vi "main.vi"() -> ()   [LabVIEW 2019]
uses:
  <vilib>/Analysis/3filter.llb/Filter Passband Type.ctl
  <vilib>/addons/control/pid/autopid.llb/PID autotuning parameters (FO).ctl
  <vilib>/Analysis/3filter.llb/Butterworth Filter (DBL).vi
  <vilib>/addons/control/pid/NI_PID_autopid.lvlib
  <vilib>/Analysis/NI_AALBase.lvlib
panel:
  in  "fine-tuning threshold (degreeC)":dbl format="%#_13g"
  in  "fine-tuning voltage (V)":dbl format="%#_13g"
  in  "limiting current (A)":dbl format="%#_13g"
  in  "heating voltage (V)":dbl format="%#_13g"
  out "Running?":bool
  in  "Graph Tab":T1(tab)
  out "Temperature Difference (sample - ambient)":cluster{dbl[], dbl[]}(graph)
  out "Temperature":cluster{dbl[], dbl[]}[](graph)
  out "Transient Power":cluster{dbl[], dbl[]}(graph)
  out "Current":cluster{dbl[], dbl[]}(graph)
  out "Voltage":cluster{dbl[], dbl[]}(graph)
  out "compensation":dbl(graph)
  out "Vp":dbl(graph)
  in  "display duration (s)":dbl format="%#_13g"
  in  "sampling interval (s)":dbl format="%#_13g"
  in  "pld_3605":refnum<visa-resource-name>
  in  "keithley_6510":refnum<visa-resource-name>
  in  "Stop Button":bool
  in  "Run Button":bool
  # "white: sample, red: ambient"
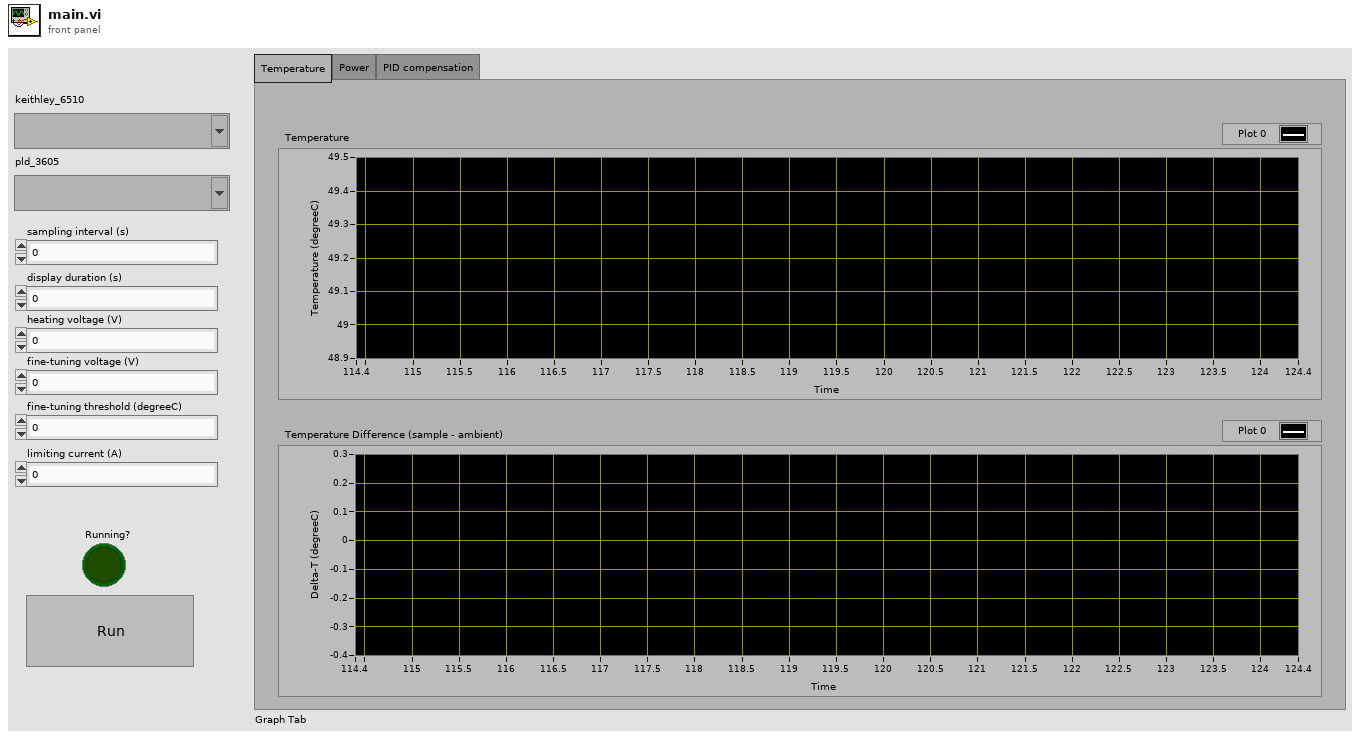
[diagram p1: front panel]
types:
  T1 = enum32{"Temperature", "Power", "PID compensation"}
  T2 = enum8{"Enabled", "Disabled", "Disabled and Grayed Out"}
  T3 = enum16{"open", "replace", "create", "open or create", "replace or create", "replace or create with confirmation"}
  T4 = cluster{"proportional gain (Kc)":dbl, "integral time (Ti, min)":dbl, "derivative time (Td, min)":dbl}
  T5 = typedef "NI_PID_autopid.lvlib/PID autotuning parameters (FO).ctl" = cluster{"type of controller":u16, "time constant factor":dbl, "step amplitude":dbl}
  T6 = typedef "NI_AALBase.lvlib/Filter Passband Type.ctl" = enum32{"Lowpass", "Highpass", "Bandpass", "Bandstop"}
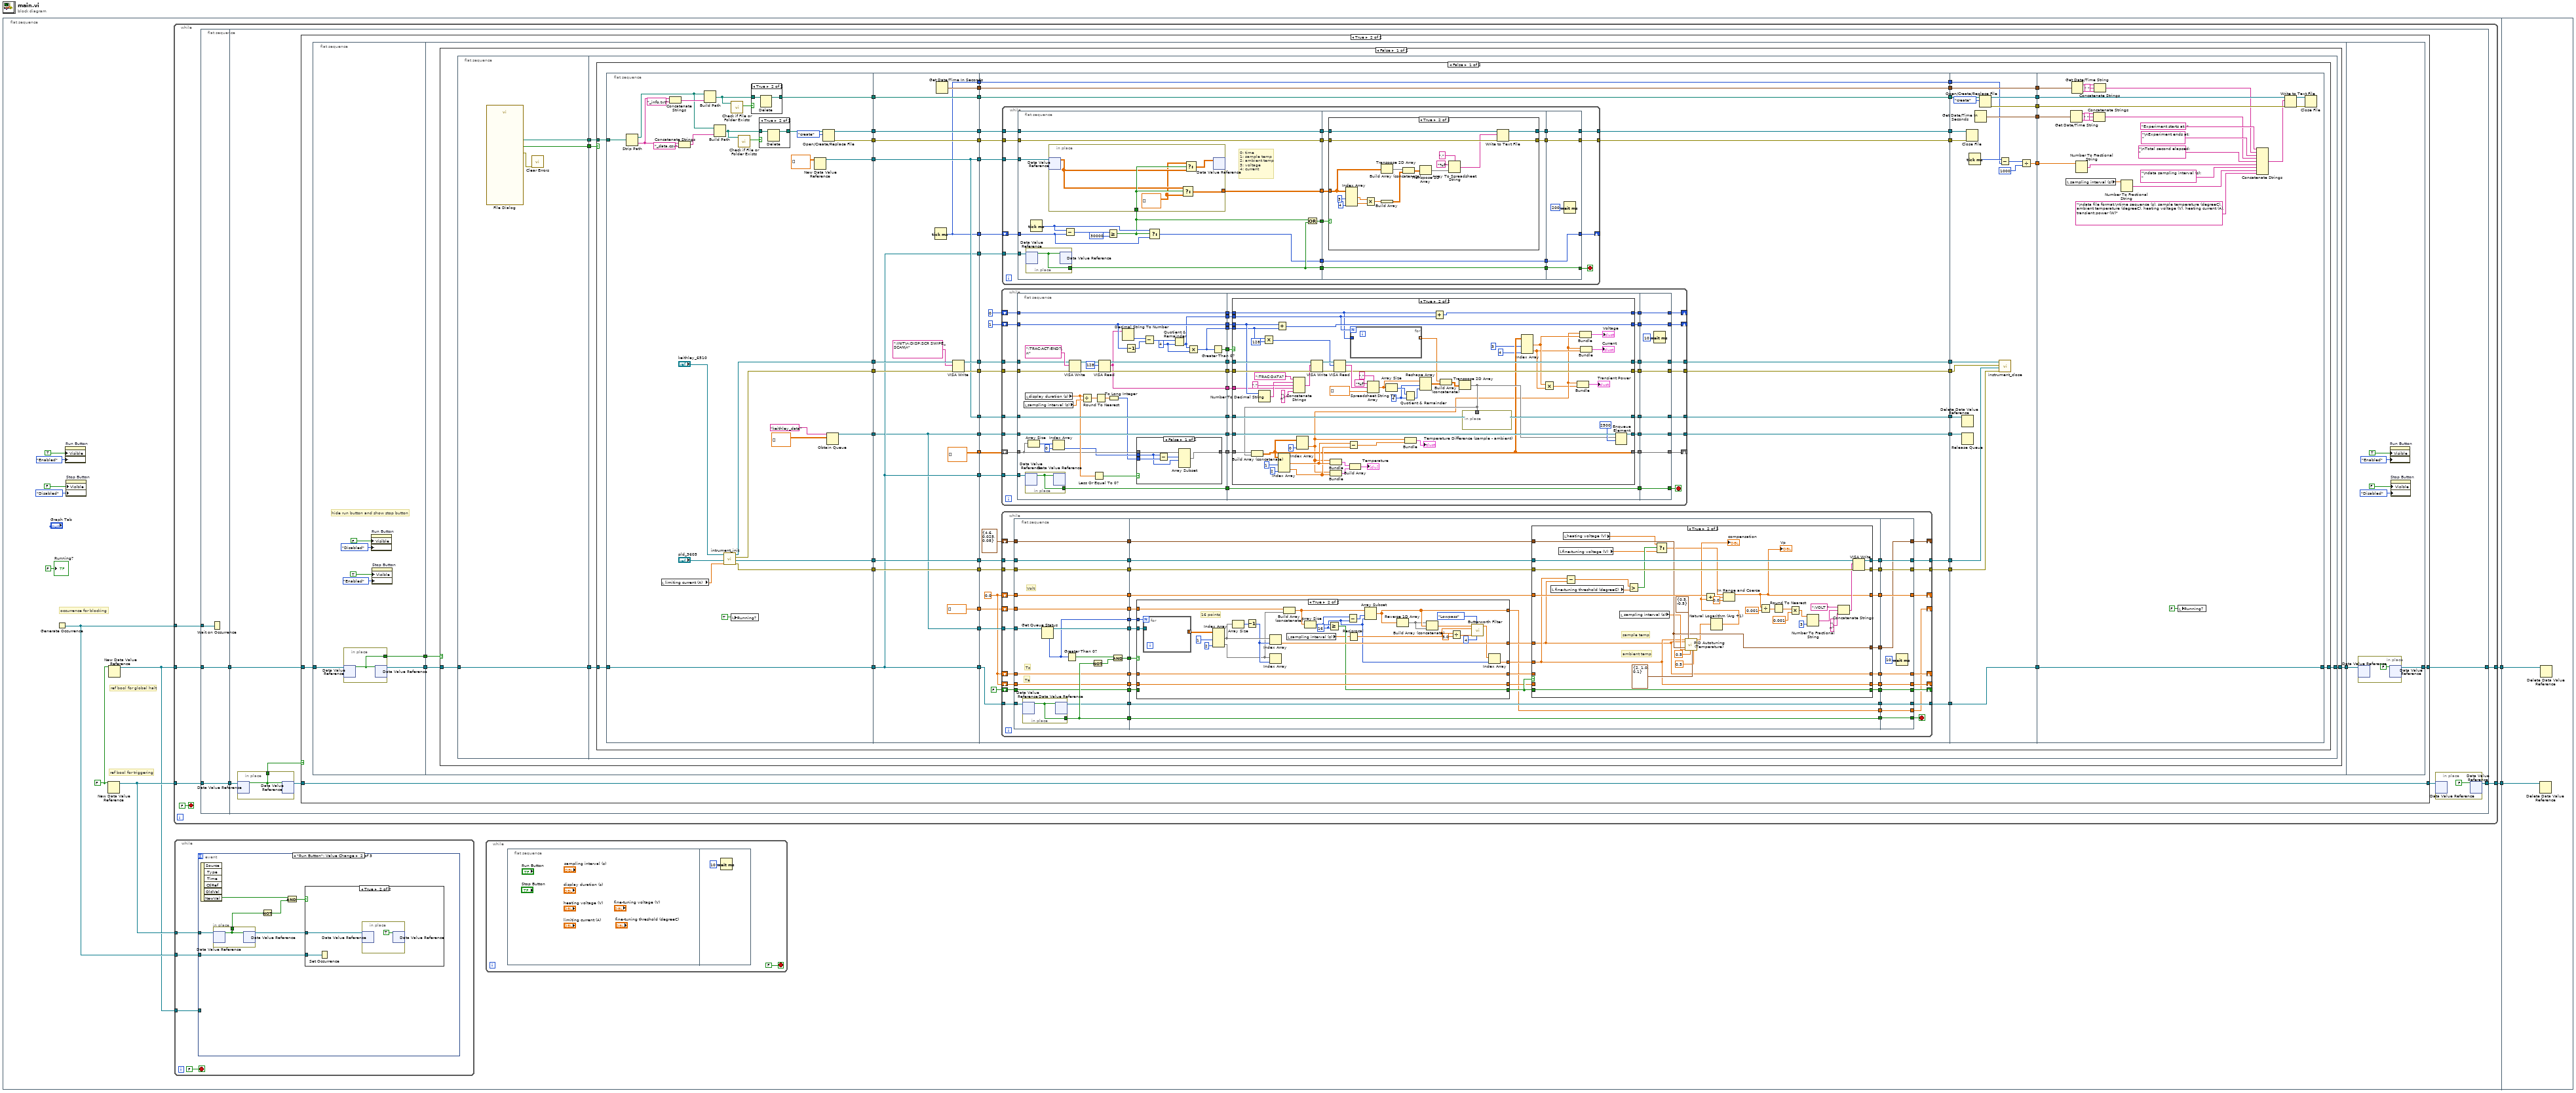
[diagram p0: block diagram]
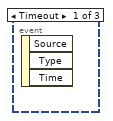
[diagram p2: hidden frame]
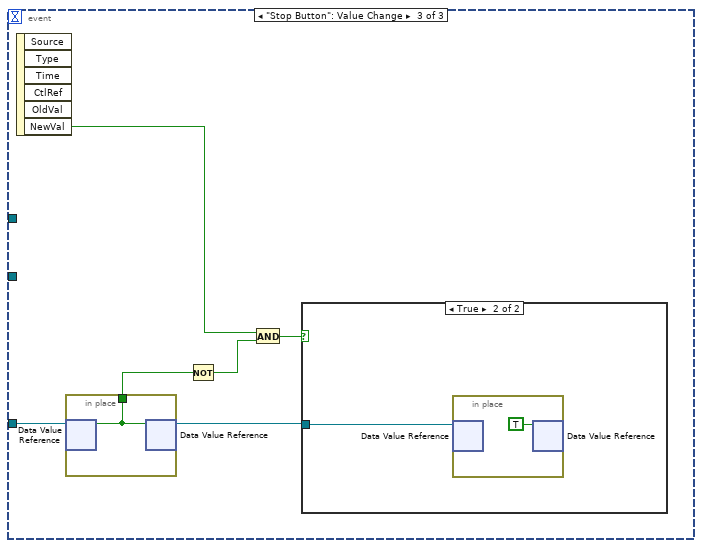
[diagram p4: hidden frame]
diagram:
  n1 = flat-sequence {
    tunnel: [w9] -> w2
    tunnel: [w8] -> w1
    tunnel: w2 -> [w706]
    tunnel: w1 -> [w705]
    frame #0 {
      w12 = FALSE
      # "occurrence for blocking"
      # "ref bool for global halt"
      # "ref bool for triggering"
      n2 = Generate Occurrence() -> (w11:refnum<k4>)
      n3 = property on="Run Button" class="Bool"("Visible"=TRUE, "DisabledEnum"=T2."Enabled" ("Disabled")) -> ()  [unwired: 2 in, 2 out]
      n4 = property on="Stop Button" class="Bool"("Visible"=FALSE, "DisabledEnum"=T2."Disabled" ("Disabled")) -> ()  [unwired: 2 in, 2 out]
      n5 = New Data Value Reference(data value=w12) -> (data value reference=w13:refnum<data-value>)  [unwired: 1 in, 1 out]
      n6 = New Data Value Reference(data value=w12) -> (data value reference=w10:refnum<data-value>)  [unwired: 1 in, 1 out]
      n7 = while {
        tunnel: w13 -> [w45]
        tunnel: w10 -> [w43]
        tunnel: w11 -> [w42]
        tunnel: [w41] -> w9
        tunnel: [w40] -> w8
        stop <- FALSE stop-if-true
        n8 = flat-sequence {
          tunnel: [w50] -> w46
          tunnel: w45 -> [w50]
          tunnel: [w49] -> w44
          tunnel: w43 -> [w49]
          tunnel: w42 -> [w48]
          tunnel: w46 -> [w57]
          tunnel: w44 -> [w55]
          tunnel: [w52] -> w41
          tunnel: [w51] -> w40
          frame #0 {
            n9 = Wait on Occurrence(2:w48) -> ()  [unwired: 2 in, 1 out]
          }
          frame #1 {
            n10 = in-place {
              in-place-border: [w59] -> w56
              n11 = in-place-dvr #1(w57) -> (w59:bool)  [unwired: 1 out]
              n12 = in-place-dvr #1(w59) -> (w54:refnum<data-value>)  [unwired: 1 out]
            }
            n13 = case shown="True" w56 {
              tunnel: w55 -> [w60 w67]
              tunnel: w54 -> [w61 w63]
              tunnel: [w61 w63] -> w53
              tunnel: [w60 w62] -> w52
              frame False {
              }
              frame True {
                n14 = flat-sequence {
                  tunnel: w67 -> [w74]
                  tunnel: [w73] -> w66
                  tunnel: [w72] -> w65
                  tunnel: w66 -> [w78]
                  tunnel: w65 -> [w77]
                  tunnel: [w76] -> w64
                  tunnel: w64 -> [w703]
                  tunnel: [w702] -> w62
                  frame #0 {
                    # "hide run button and show stop button"
                    n15 = in-place {
                      in-place-border: [w75] -> w72
                      n16 = in-place-dvr #2(w74) -> (w75:bool)  [unwired: 1 out]
                      n17 = in-place-dvr #2(w75) -> (w73:refnum<data-value>)  [unwired: 1 out]
                    }
                    n18 = property on="Run Button" class="Bool"("Visible"=FALSE, "DisabledEnum"=T2."Disabled" ("Disabled")) -> ()  [unwired: 2 in, 2 out]
                    n19 = property on="Stop Button" class="Bool"("Visible"=TRUE, "DisabledEnum"=T2."Enabled" ("Disabled")) -> ()  [unwired: 2 in, 2 out]
                  }
                  frame #1 {
                    n20 = case shown="False" w77 {
                      tunnel: w78 -> [w80 w697]
                      tunnel: [w79 w697] -> w76
                      frame False {
                        n21 = flat-sequence {
                          tunnel: [w86] -> w83
                          tunnel: [w85] -> w82
                          tunnel: [w84] -> w81
                          tunnel: w80 -> [w84]
                          tunnel: w83 -> [w91]
                          tunnel: w82 -> [w90]
                          tunnel: w81 -> [w89]
                          tunnel: [w88] -> w79
                          frame #0 {
                            n22 = call "File Dialog"() -> ("selected path"=w85:path, "cancelled"=w86:bool, "error out"=w87:errorcluster)  [unwired: 12 in, 1 out]
                            n23 = call <vilib>:"Clear Errors.vi"("error in (no error)"=w87) -> ()  [unwired: 5 in, 2 out]
                          }
                          frame #1 {
                            n24 = case shown="False" w91 {
                              tunnel: w90 -> [w141 _]
                              tunnel: w89 -> [w128 w696]
                              tunnel: [w106 w696] -> w88
                              frame False {
                                n25 = flat-sequence {
                                tunnel: w141 -> [w161]
                                tunnel: [w169] -> w139
                                tunnel: [w168] -> w138
                                tunnel: [w167] -> w137
                                tunnel: [w166] -> w136
                                tunnel: [w155] -> w135
                                tunnel: [w152] -> w133
                                tunnel: [w151] -> w132
                                tunnel: [w149] -> w131
                                tunnel: w128 -> [w148]
                                tunnel: [w148] -> w127
                                tunnel: [w145] -> w117
                                tunnel: [w193] -> w140
                                tunnel: w139 -> [w190]
                                tunnel: w138 -> [w184]
                                tunnel: w137 -> [w189]
                                tunnel: w136 -> [w183]
                                tunnel: w135 -> [w194]
                                tunnel: [w194] -> w134
                                tunnel: w133 -> [w192]
                                tunnel: w132 -> [w191]
                                tunnel: w131 -> [w185]
                                tunnel: [w192] -> w130
                                tunnel: [w191] -> w129
                                tunnel: w127 -> [w182]
                                tunnel: [w182] -> w126
                                tunnel: [w185] -> w125
                                tunnel: [w179] -> w124
                                tunnel: [w187] -> w123
                                tunnel: [w186] -> w122
                                tunnel: [w182] -> w121
                                tunnel: [w185] -> w118
                                tunnel: w117 -> [w181]
                                tunnel: [w181] -> w116
                                tunnel: [w184] -> w113
                                tunnel: [w183] -> w112
                                tunnel: [w182] -> w111
                                tunnel: [w181] -> w110
                                tunnel: [dbl[][] []] -> w96
                                tunnel: [w179] -> w95
                                tunnel: [dbl[] []] -> w92
                                tunnel: w140 -> [w200]
                                tunnel: w134 -> [w199]
                                tunnel: w130 -> [w227]
                                tunnel: w129 -> [w226]
                                tunnel: w126 -> [w225]
                                tunnel: w125 -> [w224]
                                tunnel: w124 -> [w223]
                                tunnel: w123 -> [w222]
                                tunnel: w122 -> [w221]
                                tunnel: w121 -> [w220]
                                tunnel: [w217] -> w120
                                tunnel: [w216] -> w119
                                tunnel: w118 -> [w215]
                                tunnel: w116 -> [w214]
                                tunnel: [w213] -> w115
                                tunnel: [w212] -> w114
                                tunnel: w113 -> [w211]
                                tunnel: w112 -> [w210]
                                tunnel: w111 -> [w209]
                                tunnel: w110 -> [w208]
                                tunnel: [w207] -> w109
                                tunnel: [w206] -> w108
                                tunnel: [w203] -> w107
                                tunnel: [w202] -> w104
                                tunnel: [w201] -> w103
                                tunnel: [w200] -> w102
                                tunnel: [w199] -> w101
                                tunnel: w96 -> [w198]
                                tunnel: w95 -> [w197]
                                tunnel: [w197] -> w94
                                tunnel: w92 -> [w195]
                                tunnel: w120 -> [w667]
                                tunnel: w119 -> [w666]
                                tunnel: w115 -> [w668]
                                tunnel: w114 -> [w669]
                                tunnel: w109 -> [w665]
                                tunnel: w108 -> [w664]
                                tunnel: w107 -> [w663]
                                tunnel: [w663] -> w105
                                tunnel: w104 -> [w662]
                                tunnel: w103 -> [w661]
                                tunnel: w102 -> [w659]
                                tunnel: w101 -> [w658]
                                tunnel: [w660] -> w100
                                tunnel: [w659] -> w99
                                tunnel: [w656] -> w98
                                tunnel: [w655] -> w97
                                tunnel: w94 -> [w653]
                                tunnel: [w650] -> w93
                                tunnel: [w695] -> w106
                                tunnel: w105 -> [w695]
                                tunnel: w100 -> [w683]
                                tunnel: w99 -> [w689]
                                tunnel: w98 -> [w694]
                                tunnel: w97 -> [w693]
                                tunnel: w93 -> [w671]
                                frame #0 {
                                n26 = Strip Path(path=w161) -> (stripped path=w143:path, name=w163:string)
                                n27 = local read "limiting current (A)"() -> (w142:dbl)
                                n28 = Concatenate Strings(w163, "_info.txt" ("string")) -> (w160:string)
                                n29 = Concatenate Strings(w163, "_data.csv" ("string")) -> (w162:string)
                                n30 = Build Path(base path=w143, name or relative path=w160) -> (appended path=w158:path)
                                n31 = Build Path(base path=w143, name or relative path=w162) -> (appended path=w156:path)
                                n32 = call "intrument_init.vi"("limiting current"=w142, "pld_3605_visa_input"="pld_3605", "keithley_6510_visa_input"="keithley_6510") -> ("pld_3605_error_output"=w166:errorcluster, "pld_3605_visa_output"=w168:refnum<visa-resource-name>, "keithley_6510_error_output"=w167:errorcluster, "keithley_6510_visa_output"=w169:refnum<visa-resource-name>)  [unwired: 5 in]
                                n33 = local write "Running?"(TRUE ("Running?")) -> ()
                                n34 = call <vilib>:"Check if File or Folder Exists.vi"("path"=w158) -> ("file or folder exists?"=w159:bool)  [unwired: 8 in, 2 out]
                                n35 = call <vilib>:"Check if File or Folder Exists.vi"("path"=w156) -> ("file or folder exists?"=w157:bool)  [unwired: 8 in, 2 out]
                                n36 = case shown="True" w159 {
                                tunnel: w158 -> [w175 w177]
                                tunnel: [w175 w176] -> w155
                                frame False {
                                }
                                frame True {
                                n37 = Delete(path (use dialog)=w177) -> (deleted path=w176:path)  [unwired: 4 in, 2 out]
                                }
                                }
                                n38 = case shown="True" w157 {
                                tunnel: w156 -> [w172 w174]
                                tunnel: [w172 w173] -> w154
                                frame False {
                                }
                                frame True {
                                n39 = Delete(path (use dialog)=w174) -> (deleted path=w173:path)  [unwired: 4 in, 2 out]
                                }
                                }
                                n40 = New Data Value Reference(data value=dbl[][] []) -> (data value reference=w149:refnum<data-value>)  [unwired: 1 in, 1 out]
                                n41 = Open/Create/Replace File(file path (use dialog)=w154, operation (0:open)=T3."create") -> (refnum out=w152:refnum<file>, error out=w151:errorcluster)  [unwired: 4 in, 1 out]
                                n42 = Obtain Queue(name (unnamed)="keithley_data", element data type=dbl[][] []) -> (queue out=w145:refnum<queue>)  [unwired: 3 in, 2 out]
                                }
                                frame #1 {
                                n43 = Tick Count (ms)() -> (millisecond timer value=w179:u32)
                                n44 = Get Date/Time In Seconds() -> (seconds since 1Jan1904=w193:timestamp)
                                n45 = VISA Write(VISA resource name=w190, write buffer=":INIT\n:DISP:SCR SWIPE_SCAN\n", error in (no error)=w189) -> (VISA resource name out=w187:refnum<visa-resource-name>, error out=w186:errorcluster)  [unwired: 1 out]
                                }
                                frame #2 {
                                w204 = 0.0
                                n46 = while {
                                tunnel: w222 -> [w438]
                                tunnel: w221 -> [w437]
                                tunnel: w220 -> [w436]
                                shift-right: [w430] -> _
                                shift-left: 1 -> [w435]
                                shift-right: [w417] -> _
                                shift-left: 0 -> [w421]
                                tunnel: [w416] -> w217
                                tunnel: [w415] -> w216
                                tunnel: w215 -> [w414]
                                tunnel: w214 -> [w412]
                                tunnel: [w409] -> w213
                                tunnel: [w407] -> w212
                                shift-right: [w403] -> _
                                shift-left: w198 -> [w406]
                                stop <- w427 stop-if-true
                                n47 = flat-sequence {
                                tunnel: w438 -> [w466]
                                tunnel: w437 -> [w465]
                                tunnel: w436 -> [w471]
                                tunnel: w435 -> [w459]
                                tunnel: [w460] -> w434
                                tunnel: [w459] -> w433
                                tunnel: [w458] -> w432
                                tunnel: [w457] -> w429
                                tunnel: [w456] -> w426
                                tunnel: [w455] -> w425
                                tunnel: [w454] -> w424
                                tunnel: w421 -> [w453]
                                tunnel: [w453] -> w420
                                tunnel: [w452] -> w419
                                tunnel: w414 -> [w451]
                                tunnel: [w451] -> w413
                                tunnel: w412 -> [w450]
                                tunnel: [w450] -> w411
                                tunnel: w406 -> [w444]
                                tunnel: [w439] -> w405
                                tunnel: w434 -> [w494]
                                tunnel: w433 -> [w497]
                                tunnel: w432 -> [w496]
                                tunnel: [w495] -> w431
                                tunnel: w429 -> [w493]
                                tunnel: [w493] -> w428
                                tunnel: w426 -> [w492]
                                tunnel: w425 -> [w491]
                                tunnel: w424 -> [w490]
                                tunnel: [w489] -> w423
                                tunnel: [w488] -> w422
                                tunnel: w420 -> [w487]
                                tunnel: w419 -> [w486]
                                tunnel: [w485] -> w418
                                tunnel: w413 -> [w484]
                                tunnel: w411 -> [w483]
                                tunnel: [w482] -> w410
                                tunnel: [w481] -> w408
                                tunnel: w405 -> [w480]
                                tunnel: [w479] -> w404
                                tunnel: w431 -> [w579]
                                tunnel: [w579] -> w430
                                tunnel: w428 -> [w578]
                                tunnel: [w578] -> w427
                                tunnel: w423 -> [w575]
                                tunnel: w422 -> [w574]
                                tunnel: [w576] -> w417
                                tunnel: w418 -> [w576]
                                tunnel: [w575] -> w416
                                tunnel: [w574] -> w415
                                tunnel: [w573] -> w409
                                tunnel: w410 -> [w573]
                                tunnel: w408 -> [w572]
                                tunnel: [w572] -> w407
                                tunnel: w404 -> [w571]
                                tunnel: [w571] -> w403
                                frame #0 {
                                w461 = 4 ("y")
                                n48 = local read "sampling interval (s)"() -> (w449:dbl)
                                n49 = local read "display duration (s)"() -> (w445:dbl)
                                n50 = in-place {
                                in-place-border: [w478] -> w457
                                n51 = in-place-dvr #3(w471) -> (w478:bool)  [unwired: 1 out]
                                n52 = in-place-dvr #3(w478) -> ()  [unwired: 2 out]
                                }
                                n53 = Array Size(array=w444) -> (size(s)=w443:i32[])
                                n54 = Index Array(array=w443, index=0) -> (element=w441:i32)
                                n55 = VISA Write(VISA resource name=w466, write buffer=":TRAC:ACT:END?\n", error in (no error)=w465) -> (VISA resource name out=w470:refnum<visa-resource-name>, error out=w469:errorcluster)  [unwired: 1 out]
                                n56 = Divide(x=w445, y=w449) -> (x/y=w448:dbl)
                                n57 = Less Or Equal To 0?(x=w445) -> (x <= 0?=w446:bool)
                                n58 = Round To Nearest(number=w448) -> (nearest integer value=w447:dbl)
                                n59 = VISA Read(VISA resource name=w470, byte count=u32 128, error in (no error)=w469) -> (VISA resource name out=w456:refnum<visa-resource-name>, read buffer=w454:string, error out=w455:errorcluster)  [unwired: 1 out]
                                n60 = To Long Integer(number=w447) -> (32bit integer=w440:i32)
                                n61 = Decimal String To Number(string=w454) -> (number=w464:i32)  [unwired: 2 in, 1 out]
                                n62 = Decrement(x=w459) -> (x-1=w463:i32)
                                n63 = case shown="False" w446 {
                                tunnel: w444 -> [w475 w477]
                                tunnel: w441 -> [w473 _]
                                tunnel: w440 -> [w476 _]
                                tunnel: [w472 w477] -> w439
                                frame False {
                                n64 = Subtract(x=w473, y=w476) -> (x-y=w474:i32)
                                n65 = Array Subset(array=w475, index (row)=w474, length (row)=w473) -> (w472:dbl[][])  [unwired: 2 in]
                                }
                                frame True {
                                }
                                }
                                n66 = Subtract(x=w464, y=w463) -> (x-y=w462:i32)
                                n67 = Quotient & Remainder(x=w462, y=w461) -> (floor(x/y)=w452:i32)  [unwired: 1 out]
                                n68 = Multiply(x=w452, y=w461) -> (x*y=w458:i32)
                                n69 = Greater Than 0?(x=w458) -> (x > 0?=w460:bool)
                                }
                                frame #1 {
                                n70 = case shown="True" w494 {
                                tunnel: w497 -> [w504 w555]
                                tunnel: w496 -> [_ w552]
                                tunnel: [w504 w562] -> w495
                                tunnel: w492 -> [w503 w561]
                                tunnel: w491 -> [w502 w560]
                                tunnel: w490 -> [_ w554]
                                tunnel: [w503 w539] -> w489
                                tunnel: [w502 w538] -> w488
                                tunnel: w487 -> [w501 w535]
                                tunnel: w486 -> [_ w536]
                                tunnel: [w501 w537] -> w485
                                tunnel: w484 -> [w499 w534]
                                tunnel: w483 -> [w500 w532]
                                tunnel: [w500 w530] -> w482
                                tunnel: [w499 w533] -> w481
                                tunnel: w480 -> [w498 w529]
                                tunnel: [w498 w517] -> w479
                                frame False {
                                }
                                frame True {
                                w542 = 4 ("dimension size")
                                n71 = Number To Decimal String(number=w555) -> (decimal integer string=w556:string)  [unwired: 1 in]
                                n72 = Multiply(x=w552, y=128) -> (x*y=w548:i32)
                                n73 = Add(x=w555, y=w552) -> (x+y=w562:i32)
                                n74 = Concatenate Strings(":TRAC:DATA? " ("string"), w556, "," ("string"), w554, "\n" ("string")) -> (w553:string)
                                n75 = VISA Write(VISA resource name=w561, write buffer=w553, error in (no error)=w560) -> (VISA resource name out=w550:refnum<visa-resource-name>, error out=w549:errorcluster)  [unwired: 1 out]
                                n76 = VISA Read(VISA resource name=w550, byte count=w548, error in (no error)=w549) -> (VISA resource name out=w539:refnum<visa-resource-name>, read buffer=w544:string, error out=w538:errorcluster)  [unwired: 1 out]
                                n77 = for {
                                N: w536 -> [_]
                                tunnel: w535 -> [w570]
                                tunnel: [w566] -> w506 mode=indexing
                                i -> [w569]
                                n78 = local read "sampling interval (s)"() -> (w568:dbl)
                                n79 = Add(x=w569, y=w570) -> (x+y=w567:i32)
                                n80 = Multiply(x=w567, y=w568) -> (x*y=w566:dbl)
                                }
                                n81 = Spreadsheet String To Array(delimiter (Tab)=",", format string="%f", spreadsheet string=w544, array type (2D Dbl)=dbl[] []) -> (array=w540:dbl[])
                                n82 = Array Size(array=w540) -> (size(s)=w543:i32)
                                n83 = Quotient & Remainder(x=w543, y=w542) -> (floor(x/y)=w541:i32)  [unwired: 1 out]
                                n84 = Reshape Array(w540, w542, w541) -> (w507:dbl[][])
                                n85 = Add(x=w535, y=w536) -> (x+y=w537:i32)
                                n86 = Build Array (concatenate)(w506, w507) -> (w505:dbl[][])
                                n87 = Transpose 2D Array(2D array=w505) -> (transposed array=w528:dbl[][])
                                n88 = Build Array (concatenate)(w529, w528) -> (w517:dbl[][])
                                n89 = Index Array(array=w517, index (col) #1=1 ("disabled index (col)"), index (col) #2=2 ("index (col)")) -> (element #1=w520:dbl[], element #2=w519:dbl[])  [unwired: 2 in]
                                n90 = Index Array(array=w517, index (col)=0) -> (element=w510:dbl[])  [unwired: 1 in]
                                n91 = Bundle(w510, w520) -> (w524:cluster{dbl[], dbl[]})  [unwired: 1 in]
                                n92 = Bundle(w510, w519) -> (w523:cluster{dbl[], dbl[]})  [unwired: 1 in]
                                n93 = Subtract(x=w520, y=w519) -> (x-y=w518:dbl[])
                                n94 = Build Array(w524, w523) -> (→"Temperature":cluster{dbl[], dbl[]}[])
                                n95 = Bundle(w510, w518) -> (→"Temperature Difference (sample - ambient)":cluster{dbl[], dbl[]})  [unwired: 1 in]
                                n96 = in-place {
                                in-place-border: w528 -> [w564]
                                n97 = in-place-dvr #4(w534) -> (w565:dbl[][])  [unwired: 1 out]
                                n98 = Build Array (concatenate)(w565, w564) -> (w563:dbl[][])
                                n99 = in-place-dvr #4(w563) -> (w533:refnum<data-value>)  [unwired: 1 out]
                                }
                                n100 = Index Array(array=w517, index (col) #1=3 ("disabled index (col)"), index (col) #2=4 ("index (col)")) -> (element #1=w512:dbl[], element #2=w511:dbl[])  [unwired: 2 in]
                                n101 = Multiply(x=w512, y=w511) -> (x*y=w508:dbl[])
                                n102 = Bundle(w510, w508) -> (→"Transient Power":cluster{dbl[], dbl[]})  [unwired: 1 in]
                                n103 = Bundle(w510, w512) -> (→"Voltage":cluster{dbl[], dbl[]})  [unwired: 1 in]
                                n104 = Bundle(w510, w511) -> (→"Current":cluster{dbl[], dbl[]})  [unwired: 1 in]
                                n105 = Enqueue Element(queue=w532, element=w528, timeout in ms (-1)=2500) -> (queue out=w530:refnum<queue>)  [unwired: 1 in, 2 out]
                                }
                                }
                                }
                                frame #2 {
                                n106 = Wait (ms)(milliseconds to wait=u32 10) -> ()  [unwired: 1 out]
                                }
                                }
                                }
                                n107 = while {
                                tunnel: w211 -> [w270]
                                tunnel: w210 -> [w269]
                                tunnel: w209 -> [w268]
                                tunnel: w208 -> [w264]
                                tunnel: [w258] -> w207
                                tunnel: [w257] -> w206
                                shift-right: [w249] -> _
                                shift-left: w204 -> [w254]
                                shift-right: [w238] -> _
                                shift-left: FALSE -> [w252]
                                shift-right: [w242] -> _
                                shift-left: w204 -> [w248]
                                shift-right: [w241] -> _
                                shift-left: w204 -> [w247]
                                tunnel: [w236] -> w203
                                shift-right: [w232] -> _
                                shift-left: T4 {"proportional gain (Kc)"=4.6, "integral time (Ti, min)"=0.025, "derivative time (Td, min)"=0.08} ("PID gains") -> [w235]
                                shift-right: [w228] -> _
                                shift-left: w195 -> [w231]
                                stop <- w265 stop-if-true
                                n108 = flat-sequence {
                                tunnel: w270 -> [w286]
                                tunnel: w269 -> [w285]
                                tunnel: w268 -> [w287]
                                tunnel: [w283] -> w267
                                tunnel: w264 -> [w284]
                                tunnel: [w286] -> w263
                                tunnel: [w285] -> w262
                                tunnel: [w280] -> w261
                                tunnel: [w279] -> w256
                                tunnel: [w278] -> w255
                                tunnel: w254 -> [w276]
                                tunnel: [w277] -> w253
                                tunnel: w252 -> [w277]
                                tunnel: [w276] -> w251
                                tunnel: w248 -> [w275]
                                tunnel: w247 -> [w274]
                                tunnel: [w275] -> w246
                                tunnel: [w274] -> w245
                                tunnel: [w273] -> w240
                                tunnel: w235 -> [w272]
                                tunnel: [w272] -> w234
                                tunnel: w231 -> [w271]
                                tunnel: [w271] -> w230
                                tunnel: w267 -> [w314]
                                tunnel: [w314] -> w266
                                tunnel: w263 -> [w309]
                                tunnel: w262 -> [w308]
                                tunnel: w261 -> [w313]
                                tunnel: [w303] -> w260
                                tunnel: [w302] -> w259
                                tunnel: w256 -> [w312]
                                tunnel: w255 -> [w311]
                                tunnel: w253 -> [w310]
                                tunnel: w251 -> [w306]
                                tunnel: [w301] -> w250
                                tunnel: w246 -> [w300]
                                tunnel: w245 -> [w299]
                                tunnel: [w296] -> w244
                                tunnel: [w295] -> w243
                                tunnel: w240 -> [w293]
                                tunnel: [w294] -> w239
                                tunnel: [w293] -> w237
                                tunnel: w234 -> [w292]
                                tunnel: [w291] -> w233
                                tunnel: w230 -> [w290]
                                tunnel: [w289] -> w229
                                tunnel: w266 -> [w401]
                                tunnel: [w401] -> w265
                                tunnel: w260 -> [w400]
                                tunnel: w259 -> [w399]
                                tunnel: [w400] -> w258
                                tunnel: [w399] -> w257
                                tunnel: w250 -> [w398]
                                tunnel: [w398] -> w249
                                tunnel: w244 -> [w397]
                                tunnel: w243 -> [w396]
                                tunnel: [w397] -> w242
                                tunnel: [w396] -> w241
                                tunnel: w239 -> [w395]
                                tunnel: [w395] -> w238
                                tunnel: [w394] -> w236
                                tunnel: w237 -> [w394]
                                tunnel: w233 -> [w393]
                                tunnel: [w393] -> w232
                                tunnel: w229 -> [w392]
                                tunnel: [w392] -> w228
                                frame #0 {
                                # "Volt"
                                # "Ta"
                                # "Ts"
                                n109 = in-place {
                                in-place-border: [w288] -> w283
                                n110 = in-place-dvr #5(w287) -> (w288:bool)  [unwired: 1 out]
                                n111 = in-place-dvr #5(w288) -> (w273:refnum<data-value>)  [unwired: 1 out]
                                }
                                n112 = Get Queue Status(queue=w284) -> (queue out=w279:refnum<queue>, # elements in queue=w278:i32)  [unwired: 2 in, 6 out]
                                n113 = Greater Than 0?(x=w278) -> (x > 0?=w281:bool)
                                n114 = Not(x=w283) -> (.not. x?=w282:bool)
                                n115 = And(x=w281, y=w282) -> (x .and. y?=w280:bool)
                                }
                                frame #1 {
                                n116 = case shown="True" w313 {
                                tunnel: w312 -> [_ w388]
                                tunnel: w311 -> [_ w389]
                                tunnel: w310 -> [w360 _]
                                tunnel: [w360 w376] -> w307
                                tunnel: [w359 w381] -> w305
                                tunnel: [w358 w361] -> w304
                                tunnel: w300 -> [w359 w380]
                                tunnel: w299 -> [w358 w379]
                                tunnel: [w359 w380] -> w298
                                tunnel: [w358 w379] -> w297
                                tunnel: w290 -> [w357 w378]
                                tunnel: [w357 w372] -> w289
                                frame False {
                                }
                                frame True {
                                w362 = 16 ("y")
                                # "16 points"
                                n117 = for {
                                N: w389 -> [_]
                                tunnel: w388 -> [w391]
                                tunnel: [w390] -> w387 mode=concatenating
                                n118 = Dequeue Element(queue=w391) -> (element=w390:dbl[][])  [unwired: 2 in, 3 out]
                                }
                                n119 = Index Array(array=w387, index (col) #1=1 ("disabled index (col)"), index (col) #2=2 ("index (col)")) -> (element #1=w384:dbl[], element #2=w377:dbl[])  [unwired: 2 in]
                                n120 = Array Size(array=w384) -> (size(s)=w383:i32)
                                n121 = Decrement(x=w383) -> (x-1=w382:i32)
                                n122 = Index Array(array=w384, index=w382) -> (element=w381:dbl)
                                n123 = Index Array(array=w377, index=w382) -> ()  [unwired: 1 out]
                                n124 = Build Array (concatenate)(w378, w377) -> (w375:dbl[])
                                n125 = local read "sampling interval (s)"() -> (w369:dbl)
                                n126 = Array Size(array=w375) -> (size(s)=w374:i32)
                                n127 = Greater Or Equal?(x=w374, y=w362) -> (x >= y?=w376:bool)
                                n128 = Subtract(x=w374, y=w362) -> (x-y=w373:i32)
                                n129 = Reciprocal(x=w369) -> (1/x=w367:dbl)
                                n130 = Array Subset(array=w375, index=w373, length=w362) -> (w372:dbl[])
                                n131 = Reverse 1D Array(array=w372) -> (reversed array=w371:dbl[])
                                n132 = Build Array (concatenate)(w371, w372, w371) -> (w370:dbl[])
                                n133 = Divide(x=w367, y=3.0) -> (x/y=w365:dbl)
                                n134 = call-poly <vilib>:"Butterworth Filter.vi"("order"=4, "filter type"=Filter_Passband_Type."Lowpass", "low cutoff freq: fl"=w365, "sampling freq: fs"=w367, "X"=w370) -> ("Filtered X"=w363:dbl[])  [unwired: 3 in, 1 out]
                                n135 = Index Array(array=w363, index=w362) -> (element=w361:dbl)
                                }
                                }
                                n136 = case shown="True" w307 {
                                tunnel: w309 -> [w321 w355]
                                tunnel: w308 -> [w320 w354]
                                tunnel: w307 -> [w316 w342]
                                tunnel: w306 -> [w319 w356]
                                tunnel: w305 -> [_ w328]
                                tunnel: w304 -> [_ w329]
                                tunnel: [w321 w353] -> w303
                                tunnel: [w320 w352] -> w302
                                tunnel: [w319 w331] -> w301
                                tunnel: w298 -> [w318 _]
                                tunnel: w297 -> [w317 _]
                                tunnel: [w318 w328] -> w296
                                tunnel: [w317 w329] -> w295
                                tunnel: [w316 w342] -> w294
                                tunnel: w292 -> [w315 w334]
                                tunnel: [w315 w334] -> w291
                                frame False {
                                }
                                frame True {
                                # "ambient temp"
                                # "sample temp"
                                n137 = local read "fine-tuning threshold (degreeC)"() -> (w326:dbl)
                                n138 = local read "fine-tuning voltage (V)"() -> (w323:dbl)
                                n139 = local read "heating voltage (V)"() -> (w324:dbl)
                                n140 = Subtract(x=w329, y=w328) -> (x-y=w327:dbl)
                                n141 = local read "sampling interval (s)"() -> (w330:dbl)
                                n142 = Greater?(x=w327, y=w326) -> (0:w325:bool)
                                n143 = Select(t=w324, s=w325, f=w323) -> (s? t:f=w322:dbl)
                                n144 = call <vilib>:"PID Autotuning (Temperature).vi"("desired temperature"=w329, "measured temperature"=w328, "PID gains in"=w334, "dt (s)"=w330, "output range"=cluster{"output high":dbl, "output low":dbl} {"output high"=0.5, "output low"=-0.5}, "beta"=0.5, "autotuning parameters"=T5 {"type of controller"=2, "time constant factor"=1.0, "step amplitude"=0.1}, "alpha"=0.5) -> ("output"=w333:dbl)  [unwired: 8 in, 3 out]
                                n145 = Natural Logarithm (Arg +1)(1:w333) -> (0:w332:dbl)
                                "compensation" <- w332
                                n146 = Add(x=w356, y=w332) -> (x+y=w339:dbl)
                                n147 = In Range and Coerce(upper limit=w322, x=w339, lower limit=0.0) -> (coerced(x)=w331:dbl)  [unwired: 1 out]
                                "Vp" <- w331
                                n148 = Divide(x=w331, y=0.001) -> (x/y=w350:dbl)
                                n149 = Round To Nearest(number=w350) -> (nearest integer value=w349:dbl)
                                n150 = Multiply(x=w349, y=0.001) -> (x*y=w345:dbl)
                                n151 = Number To Fractional String(number=w345, precision (6)=i16 3) -> (F-format string=w344:string)  [unwired: 2 in]
                                n152 = Concatenate Strings(":VOLT " ("write buffer"), w344, "\n" ("string")) -> (w341:string)
                                n153 = VISA Write(VISA resource name=w355, write buffer=w341, error in (no error)=w354) -> (VISA resource name out=w353:refnum<visa-resource-name>, error out=w352:errorcluster)  [unwired: 1 out]
                                }
                                }
                                }
                                frame #2 {
                                n154 = Wait (ms)(milliseconds to wait=u32 10) -> ()  [unwired: 1 out]
                                }
                                }
                                }
                                n155 = while {
                                tunnel: w227 -> [w598]
                                tunnel: w226 -> [w597]
                                tunnel: w225 -> [w596]
                                tunnel: w224 -> [w595]
                                shift-right: [w588] -> _
                                shift-left: w223 -> [w591]
                                tunnel: [w581] -> w202
                                tunnel: [w580] -> w201
                                stop <- w592 stop-if-true
                                n156 = flat-sequence {
                                tunnel: w598 -> [w602]
                                tunnel: w597 -> [w601]
                                tunnel: w596 -> [w611]
                                tunnel: w595 -> [w609]
                                tunnel: [w610] -> w594
                                tunnel: w591 -> [w605]
                                tunnel: [w604] -> w590
                                tunnel: [w603] -> w587
                                tunnel: [w602] -> w586
                                tunnel: [w601] -> w585
                                tunnel: [w599] -> w584
                                tunnel: w594 -> [w625]
                                tunnel: [w625] -> w593
                                tunnel: w590 -> [w624]
                                tunnel: [w624] -> w589
                                tunnel: w587 -> [w623]
                                tunnel: w586 -> [w622]
                                tunnel: w585 -> [w621]
                                tunnel: w584 -> [w620]
                                tunnel: [w619] -> w583
                                tunnel: [w618] -> w582
                                tunnel: w593 -> [w648]
                                tunnel: [w648] -> w592
                                tunnel: w589 -> [w647]
                                tunnel: [w647] -> w588
                                tunnel: w583 -> [w646]
                                tunnel: w582 -> [w645]
                                tunnel: [w646] -> w581
                                tunnel: [w645] -> w580
                                frame #0 {
                                # "0: time\n1: sample temp\n2: ambient temp\n3: voltage\n4: current"
                                n157 = in-place {
                                in-place-border: [w617] -> w610
                                n158 = in-place-dvr #6(w611) -> (w617:bool)  [unwired: 1 out]
                                n159 = in-place-dvr #6(w617) -> ()  [unwired: 2 out]
                                }
                                n160 = Tick Count (ms)() -> (millisecond timer value=w606:u32)
                                n161 = Subtract(x=w606, y=w605) -> (x-y=w608:u32)
                                n162 = Greater Or Equal?(x=w608, y=u32 30000) -> (x >= y?=w600:bool)
                                n163 = in-place {
                                in-place-border: w600 -> [w616]
                                in-place-border: [w612] -> w599
                                w614 = dbl[][] [] ("f")
                                n164 = in-place-dvr #7(w609) -> (w615:dbl[][])  [unwired: 1 out]
                                n165 = Select(t=w615, s=w616, f=w614) -> (s? t:f=w612:dbl[][])
                                n166 = Select(t=w614, s=w616, f=w615) -> (s? t:f=w613:dbl[][])
                                n167 = in-place-dvr #7(w613) -> ()  [unwired: 2 out]
                                }
                                n168 = Select(t=w606, s=w600, f=w605) -> (s? t:f=w604:u32)
                                n169 = Or(x=w600, y=w610) -> (x .or. y?=w603:bool)
                                }
                                frame #1 {
                                n170 = case shown="True" w623 {
                                tunnel: w622 -> [w627 w644]
                                tunnel: w621 -> [w626 w643]
                                tunnel: w620 -> [_ w637]
                                tunnel: [w627 w629] -> w619
                                tunnel: [w626 w628] -> w618
                                frame False {
                                }
                                frame True {
                                n171 = Index Array(array=w637, index (col) #1=3 ("disabled index (col)"), index (col) #2=4 ("index (col)")) -> (element #1=w640:dbl[], element #2=w639:dbl[])  [unwired: 2 in]
                                n172 = Multiply(x=w640, y=w639) -> (x*y=w638:dbl[])
                                n173 = Build Array(w638) -> (w634:dbl[][])
                                n174 = Transpose 2D Array(2D array=w637) -> (transposed array=w636:dbl[][])
                                n175 = Build Array (concatenate)(w636, w634) -> (w635:dbl[][])
                                n176 = Transpose 2D Array(2D array=w635) -> (transposed array=w633:dbl[][])
                                n177 = Array To Spreadsheet String(delimiter (Tab)=",", array=w633, 3:"%f" ("format string")) -> (spreadsheet string=w630:string)
                                n178 = Write to Text File(file (use dialog)=w644, text=w630, error in=w643) -> (refnum out=w629:refnum<file>, error out=w628:errorcluster)  [unwired: 1 in, 1 out]
                                }
                                }
                                }
                                frame #2 {
                                n179 = Wait (ms)(milliseconds to wait=u32 200) -> ()  [unwired: 1 out]
                                }
                                }
                                }
                                }
                                frame #3 {
                                n180 = Delete Data Value Reference(data value reference=w669) -> ()  [unwired: 1 in, 2 out]
                                n181 = Release Queue(queue=w668) -> ()  [unwired: 2 in, 3 out]
                                n182 = Close File(refnum=w662, error in=w661) -> ()  [unwired: 2 out]
                                n183 = Tick Count (ms)() -> (millisecond timer value=w654:u32)
                                n184 = Get Date/Time In Seconds() -> (seconds since 1Jan1904=w660:timestamp)
                                n185 = Open/Create/Replace File(file path (use dialog)=w658, operation (0:open)=T3."create") -> (refnum out=w656:refnum<file>, error out=w655:errorcluster)  [unwired: 4 in, 1 out]
                                n186 = Subtract(x=w654, y=w653) -> (x-y=w652:u32)
                                n187 = call "instrument_close.vi"("pld_3605_error_input"=w664, "pld_3605"=w665, "keithley_6510_error_input"=w666, "keithley_6510"=w667) -> ()  [unwired: 8 in]
                                n188 = Divide(x=w652, y=u32 1000) -> (x/y=w650:dbl)
                                }
                                frame #4 {
                                n189 = local read "sampling interval (s)"() -> (w679:dbl)
                                n190 = Get Date/Time String(seconds (now)=w683) -> (date string=w684:string, time string=w685:string)  [unwired: 2 in]
                                n191 = Get Date/Time String(seconds (now)=w689) -> (date string=w688:string, time string=w687:string)  [unwired: 2 in]
                                n192 = Number To Fractional String(number=w671) -> (F-format string=w670:string)  [unwired: 3 in]
                                n193 = Concatenate Strings(w684, " " ("string"), w685) -> (w681:string)
                                n194 = Concatenate Strings(w688, " " ("string"), w687) -> (w686:string)
                                n195 = Number To Fractional String(number=w679) -> (F-format string=w678:string)  [unwired: 3 in]
                                n196 = local write "Running?"(FALSE ("Running?")) -> ()
                                n197 = Concatenate Strings("Experiment starts at: " ("string"), w686, "\nExperiment ends at: " ("string"), w681, "\nTotal second elapsed: " ("string"), w670, "\ndata sampling interval (s): " ("string"), w678, "\ndata file format:\ntime sequence (s), sample temperature (degreeC), ambient temperature (degreeC), heating voltage (V), heating current (A), transient power (W)" ("string")) -> (w676:string)
                                n198 = Write to Text File(file (use dialog)=w694, text=w676, error in=w693) -> (refnum out=w692:refnum<file>, error out=w691:errorcluster)  [unwired: 1 in, 1 out]
                                n199 = Close File(refnum=w692, error in=w691) -> ()  [unwired: 2 out]
                                }
                                }
                              }
                              frame True {
                              }
                            }
                          }
                        }
                      }
                      frame True {
                      }
                    }
                  }
                  frame #2 {
                    n200 = in-place {
                      n201 = in-place-dvr #8(w703) -> ()  [unwired: 2 out]
                      n202 = in-place-dvr #8(FALSE ("data value")) -> (w702:refnum<data-value>)  [unwired: 1 out]
                    }
                    n203 = property on="Run Button" class="Bool"("Visible"=TRUE, "DisabledEnum"=T2."Enabled" ("Disabled")) -> ()  [unwired: 2 in, 2 out]
                    n204 = property on="Stop Button" class="Bool"("Visible"=FALSE, "DisabledEnum"=T2."Disabled" ("Disabled")) -> ()  [unwired: 2 in, 2 out]
                  }
                }
              }
            }
            n205 = in-place {
              n206 = in-place-dvr #9(w53) -> ()  [unwired: 2 out]
              n207 = in-place-dvr #9(FALSE ("data value")) -> (w51:refnum<data-value>)  [unwired: 1 out]
            }
          }
        }
      }
      n208 = while {
        tunnel: w13 -> [w16]
        tunnel: w11 -> [w15]
        tunnel: w10 -> [w14]
        stop <- FALSE stop-if-true
        n209 = event shown="[1] \"Run Button\": Value Change" {
          selector: _ -> [_ _ _]
          dyn-events: _ -> [_ _ _]
          timeout: _ -> [_ _ _]
          tunnel: w16 -> [_ w23 _]
          tunnel: w15 -> [_ w24 _]
          tunnel: w14 -> [_ _ w31]
          event Timeout {
            n210 = event-data() -> ()  [unwired: 1 in, 3 out]
          }
          event "Run Button": Value Change {
            n211 = event-data() -> ("NewVal"=w18:bool)  [unwired: 1 in, 5 out]
            n212 = in-place {
              in-place-border: [w25] -> w19
              n213 = in-place-dvr #10(w23) -> (w25:bool)  [unwired: 1 out]
              n214 = in-place-dvr #10(w25) -> (w22:refnum<data-value>)  [unwired: 1 out]
            }
            n215 = Not(x=w19) -> (.not. x?=w20:bool)
            n216 = And(x=w18, y=w20) -> (x .and. y?=w21:bool)
            n217 = case shown="True" w21 {
              tunnel: w22 -> [_ w27]
              tunnel: w24 -> [_ w26]
              frame False {
              }
              frame True {
                n218 = Set Occurrence(w26) -> ()
                n219 = in-place {
                  n220 = in-place-dvr #11(w27) -> ()  [unwired: 2 out]
                  n221 = in-place-dvr #11(TRUE ("data value")) -> ()  [unwired: 2 out]
                }
              }
            }
          }
          event "Stop Button": Value Change {
            n222 = event-data() -> ("NewVal"=w32:bool)  [unwired: 1 in, 5 out]
            n223 = in-place {
              in-place-border: [w35] -> w29
              n224 = in-place-dvr #12(w31) -> (w35:bool)  [unwired: 1 out]
              n225 = in-place-dvr #12(w35) -> (w30:refnum<data-value>)  [unwired: 1 out]
            }
            n226 = Not(x=w29) -> (.not. x?=w33:bool)
            n227 = And(x=w32, y=w33) -> (x .and. y?=w34:bool)
            n228 = case shown="True" w34 {
              tunnel: w30 -> [_ w36]
              frame False {
              }
              frame True {
                n229 = in-place {
                  n230 = in-place-dvr #13(w36) -> ()  [unwired: 2 out]
                  n231 = in-place-dvr #13(TRUE ("data value")) -> ()  [unwired: 2 out]
                }
              }
            }
          }
        }
      }
      n232 = while {
        stop <- FALSE stop-if-true
        n233 = flat-sequence {
          frame #0 {
          }
          frame #1 {
            n234 = Wait (ms)(milliseconds to wait=u32 10) -> ()  [unwired: 1 out]
          }
        }
      }
      "Running?" <- FALSE ("Running?")
    }
    frame #1 {
      n235 = Delete Data Value Reference(data value reference=w705) -> ()  [unwired: 1 in, 2 out]
      n236 = Delete Data Value Reference(data value reference=w706) -> ()  [unwired: 1 in, 2 out]
    }
  }
